vi "SetAttributeViInt32_SA-BP_CP_PS.vi"(7 "AttributeValue":i32 format="%.0g", 8 "error in (no error)":errorcluster {"code" format="%.0x"}, 9 "AttributeID":u32(ring)=1150205 items=["SA_BURSTPOWER_AVERAGE_COUNT"=1150205, "SA_BURSTPOWER_AVERAGE_MODE"=1150207, "SA_BURSTPOWER_AVERAGE_TYPE"=1150208, "SA_BURSTPOWER_DISPLAY_WINDOWX_REF_POSITION"=1150216, "SA_BURSTPOWER_DISPLAY_WINDOWY_REF_POSITION"=1150219, "SA_BURSTPOWER_MARKER_ACTIVE_MARKER"=1150226, "SA_BURSTPOWER_MARKER_DELTA_REFERENCE"=1150245, "SA_BURSTPOWER_MARKER_TRACE"=1150247, "SA_BURSTPOWER_MARKER_TYPE"=1150231, "SA_BURSTPOWER_MEASUREMENT_METHOD"=1150195, "SA_BURSTPOWER_SWEEPCOUPLING_BANDWIDTH_SHAPE"=1150210, "SA_BURSTPOWER_THRESHOLD_TYPE"=1150198, "SA_BURSTPOWER_TRIGGER_SOURCE"=1150199, "SA_CHANNEL_POWER_PSD_UNIT"=1150865, "SA_CHANNELPOWER_AVERAGE_COUNT"=1150251, "SA_CHANNELPOWER_AVERAGE_MODE"=1150253, "SA_CHANNELPOWER_DETECTOR_TYPE"=1150248, "SA_CHANNELPOWER_DISPLAY_WINDOWY_REF_POSITION"=1150304, "SA_CHANNELPOWER_FREQUENCY_PHASE_NOISE_OPTION_STATE"=1150264, "SA_CHANNELPOWER_MARKER_ACTIVE_MARKER"=1150276, "SA_CHANNELPOWER_MARKER_DELTA_REFERENCE"=1150281, "SA_CHANNELPOWER_MARKER_TYPE"=1150284, "SA_CHANNELPOWER_SWEEPCOUPLING_BANDWIDTH_SHAPE"=1150255, "SA_CHANNELPOWER_SWEEPCOUPLING_SWEEP_POINTS"=1150271, "SA_CHANNELPOWER_SWEEPCOUPLING_SWEEP_TIME_AUTO_RULES"=1150274, "SA_CHANNELPOWER_TRACES_TYPE"=1150778, "SA_CHANNELPOWER_TRIGGER_SOURCE"=1150269, "SA_POWERSTATISTICS_MARKER_ACTIVE_MARKER"=1150345, "SA_POWERSTATISTICS_MARKER_DELTA_REFERENCE"=1150349, "SA_POWERSTATISTICS_MARKER_TRACE"=1150353, "SA_POWERSTATISTICS_MARKER_TYPE"=1150354, "SA_POWERSTATISTICS_SAMPLING_COUNT"=1150313, "SA_POWERSTATISTICS_SWEEPCOUPLING_SWEEP_CYCLES"=1150342, "SA_POWERSTATISTICS_TRIGGER_SOURCE"=1150315], 11 "instrument handle":refnum<k15>) -> (0 "error out":errorcluster {"code" format="%.0x"}, 3 "instrument handle out":refnum<k15>)   [LabVIEW 2009, in "Keysight XSAn.lvlib"]
doc: "Sets an Int32 attribute from the instrument driver.\nThe following Attributes are supported:\n\nSA_BURSTPOWER_AVERAGE_COUNT\nSA_BURSTPOWER_AVERAGE_MODE\nSA_BURSTPOWER_AVERAGE_TYPE\nSA_BURSTPOWER_DISPLAY_WINDOWX_REF_POSITION\nSA_BURSTPOWER_DISPLAY_WINDOWY_REF_POSITION\nSA_BURSTPOWER_MARKER_ACTIVE_MARKER\nSA_BURSTPOWER_MARKER_DELTA_REFERENCE\nSA_BURSTPOWER_MARKER_TRACE\nSA_BURSTPOWER_MARKER_TYPE\nSA_BURSTPOWER_MEASUREMENT_METHOD\nSA_BURSTPOWER_SWEEPCOUPLING_BANDWIDTH_SHAPE\nSA_BURSTPOWER_THRESHOLD_TYPE\nSA_BURSTPOWER_TRIGGER_SOURCE\nSA_CHANNEL_POWER_PSD_UNIT\nSA_CHANNELPOWER_AVERAGE_COUNT\nSA_CHANNELPOWER_AVERAGE_MODE\nSA_CHANNELPOWER_DETECTOR_TYPE\nSA_CHANNELPOWER_DISPLAY_WINDOWY_REF_POSITION\nSA_CHANNELPOWER_FREQUENCY_PHASE_NOISE_OPTION_STATE\nSA_CHANNELPOWER_MARKER_ACTIVE_MARKER\nSA_CHANNELPOWER_MARKER_DELTA_REFERENCE\nSA_CHANNELPOWER_MARKER_TYPE\nSA_CHANNELPOWER_SWEEPCOUPLING_BANDWIDTH_SHAPE\nSA_CHANNELPOWER_SWEEPCOUPLING_SWEEP_POINTS\nSA_CHANNELPOWER_SWEEPCOUPLING_SWEEP_TIME_AUTO_RULES\nSA_CHANNELPOWER_TRACES_TYPE\nSA_CHANNELPOWER_TRIGGER_SOURCE\nSA_POWERSTATISTICS_MARKER_ACTIVE_MARKER\nSA_POWERSTATISTICS_MARKER_DELTA_REFERENCE\nSA_POWERSTATISTICS_MARKER_TRACE\nSA_POWERSTATISTICS_MARKER_TYPE\nSA_POWERSTATISTICS_SAMPLING_COUNT\nSA_POWERSTATISTICS_SWEEPCOUPLING_SWEEP_CYCLES\nSA_POWERSTATISTICS_TRIGGER_SOURCE"
uses:
  <instrlib>/Keysight XSAn/Keysight XSAn.lvlib
  AgXSAn.dll
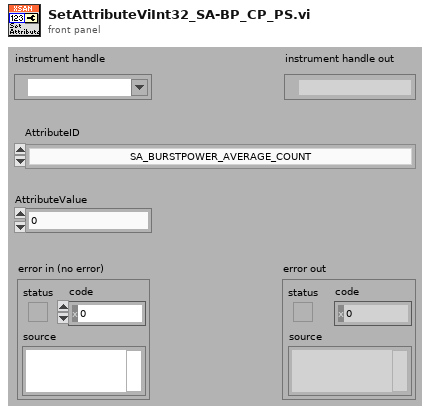
[diagram p1: front panel]
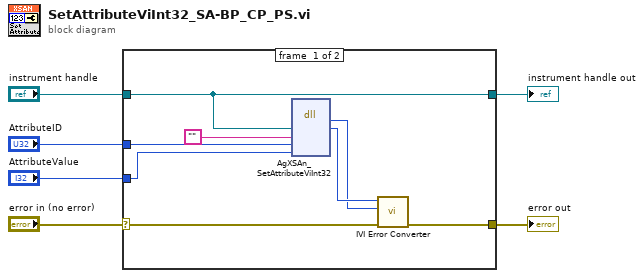
[diagram p0: block diagram]
diagram:
  n1 = case shown="No Error" "error in (no error)" {
    selector: "error in (no error)" -> [w12 w16]
    tunnel: [w11 w16] -> w6
    tunnel: "instrument handle" -> [w8 w15]
    tunnel: "AttributeID" -> [w10 _]
    tunnel: "AttributeValue" -> [w9 _]
    tunnel: [w8 w15] -> w1
    frame #0 {
      n2 = dll-call lib="AgXSAn**.dll" fn="AgXSAn_SetAttributeViInt32"("Vi"=w8, "RepCapIdentifier"="", "AttributeID"=w10, "AttributeValue"=w9) -> ("return type"=w13:i32, "Vi"=w14:u32)  [unwired: 6 in, 2 out]
      n3 = call <instrlib>:"IVI Error Converter.vi"("error in (no error)"=w12, "IVI error code (0)"=w13, "instrument handle"=w14) -> ("error out"=w11:errorcluster)  [unwired: 7 in, 1 out]
    }
    frame #1 {
    }
  }
  "error out" <- w6
  "instrument handle out" <- w1
